vi "Write Node to VIPB.vi"(8 "error in (no error)":errorcluster, 9 "New Text":string, 10 "Node Name":string, 11 "VIPB File Path":path) -> (0 "error out":errorcluster, 3 "VIPB File Path out":path)   [LabVIEW 2019, in "VIPM.lvlib"]
doc: "Returns the combined values of <B>Text_Node</B> children that the <B>node in</B> node owns."
uses:
  VIPM.lvlib
  <vilib>/regexp/Match Regular Expression.xnode
panel:
  out "result string":string
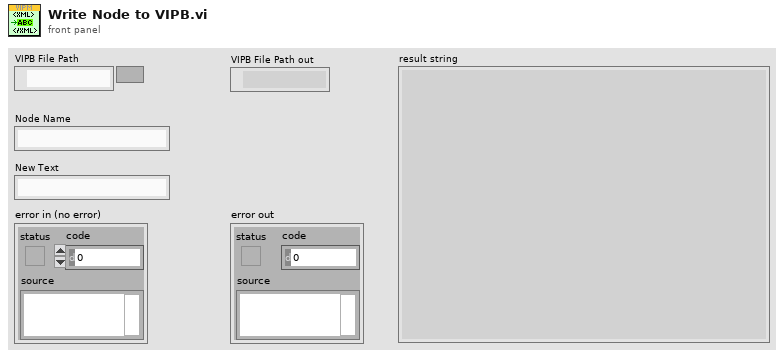
[diagram p1: front panel]
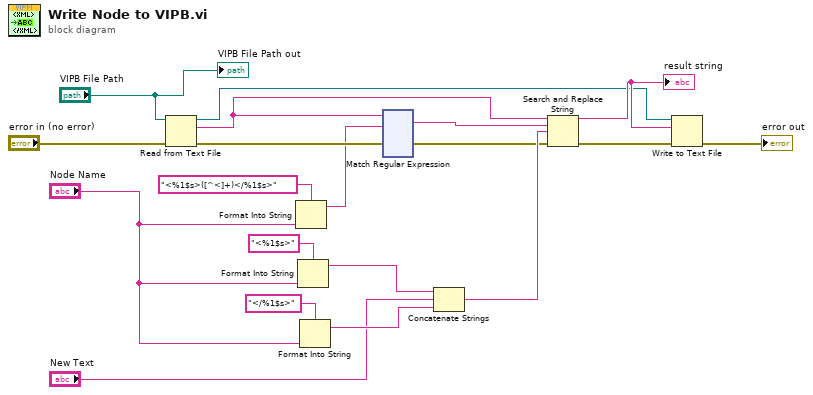
[diagram p0: block diagram]
diagram:
  n1 = Read from Text File(file (use dialog)="VIPB File Path", error in="error in (no error)") -> (refnum out=w3:refnum<file>, text=w6:string, error out=w16:errorcluster)  [unwired: 2 in, 1 out]
  n2 = Format Into String(format string="<%1$s>([^<]+)</%1$s>", "Node Name") -> (resulting string=w15:string)  [unwired: 2 in, 1 out]
  n3 = Format Into String(format string="<%1$s>", "Node Name") -> (resulting string=w11:string)  [unwired: 2 in, 1 out]
  n4 = Format Into String(format string="</%1$s>", "Node Name") -> (resulting string=w10:string)  [unwired: 2 in, 1 out]
  n5 = xnode "Match Regular Expression"("input string"=w6, "regular expression"=w15, "error in"=w16) -> ("whole match"=w12:string, "error out"=w7:errorcluster)  [unwired: 3 in, 4 out]
  n6 = Concatenate Strings(w11, "New Text", w10) -> (w8:string)
  n7 = Search and Replace String(input string=w6, search string=w12, replace string=w8, error in=w7) -> (result string=w4:string, error out=w5:errorcluster)  [unwired: 4 in, 2 out]
  "result string" <- w4
  n8 = Write to Text File(file (use dialog)=w3, text=w4, error in=w5) -> (error out=→"error out":errorcluster)  [unwired: 1 in, 2 out]
  "VIPB File Path out" <- "VIPB File Path"
